vi "new_graph.vi"(4 "CurvesId":i32, 5 "D&T":string, 7 "connection ref":T1) -> (0 "error out":errorcluster, 1 "Waveform Graph":cluster{sgl, sgl, sgl[]}, 2 "reason":string, 3 "phwnd":string[][](table))   [LabVIEW 2010]
uses:
  <vilib>/addons/database/Connection.llb/Conn ObjectReference.ctl
  <vilib>/addons/database/NI_Database_API.lvlib
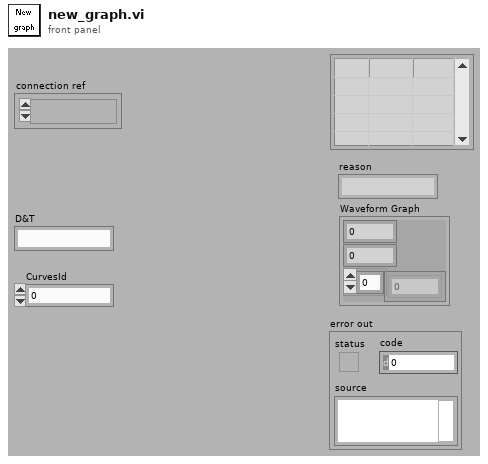
[diagram p1: front panel]
types:
  T1 = typedef "NI_Database_API.lvlib/Conn ObjectReference.ctl" = refnum<k1>
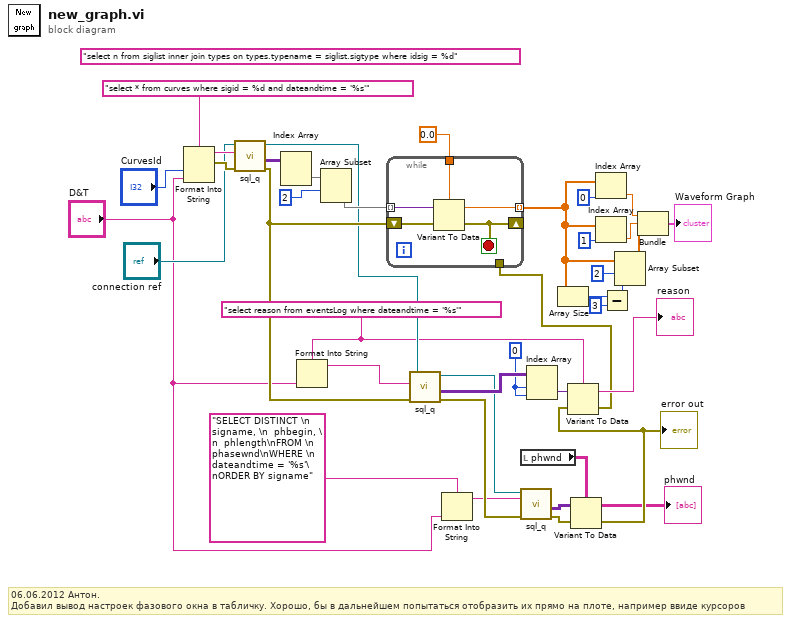
[diagram p0: block diagram]
diagram:
  w16 = 0 ("index (row)")
  w15 = "select reason from eventsLog where dateandtime = '%s'"
  (unwired) "select n from siglist inner join types on types.typename = siglist.sigtype where idsig = %d" ("regular expression (\"\")")
  # "06.06.2012 Антон. \nДобавил вывод настроек фазового окна в табличку. Хорошо, бы в дальнейшем попытаться отобразить их прямо на плоте, например ввиде курсоров"
  n1 = Format Into String(format string="select * from curves where sigid = %d and dateandtime = '%s'" ("optional clause"), "CurvesId", "D&T") -> (resulting string=w32:string, error out=w27:errorcluster)  [unwired: 2 in]
  n2 = call "sql_q.vi"("error in"=w27, "SQL query"=w32, "connect ref"="connection ref") -> ("error out"=w20:errorcluster, "recordset data"=w34:variant[][], "conn ref out"=w19:T1)  [unwired: 1 in, 1 out]
  n3 = Index Array(array=w34) -> (element=w35:variant[])  [unwired: 2 in]
  n4 = Format Into String(format string=w15, "D&T") -> (resulting string=w9:string)  [unwired: 2 in, 1 out]
  n5 = Array Subset(array=w35, index=2) -> (w33:variant[])  [unwired: 1 in]
  n6 = call "sql_q.vi"("error in"=w20, "SQL query"=w9, "connect ref"=w19) -> ("error out"=w11:errorcluster, "recordset data"=w18:variant[][], "conn ref out"=w6:T1)  [unwired: 1 in, 1 out]
  n7 = Format Into String(format string="SELECT DISTINCT \n  signame, \n  phbegin, \n  phlength\nFROM \n  phasewnd\nWHERE \n  dateandtime = '%s'\nORDER BY signame", "D&T") -> (resulting string=w7:string)  [unwired: 2 in, 1 out]
  n8 = local read "phwnd"() -> (w2:string[][])
  n9 = call "sql_q.vi"("error in"=w11, "SQL query"=w7, "connect ref"=w6) -> ("error out"=w4:errorcluster, "recordset data"=w5:variant[][])  [unwired: 1 in, 2 out]
  n10 = Index Array(array=w18, index (row)=w16, index (col)=w16) -> (element=w17:variant)
  n11 = Variant To Data(error in=w4, Variant=w5, type=w2) -> (error out=w3:errorcluster, data=→"phwnd":string[][])
  "error out" <- w3
  n12 = Variant To Data(error in=w3, Variant=w17, type=w15) -> (error out=w13:errorcluster, data=→"reason":string)
  n13 = while {
    tunnel: [w45] -> w23 mode=indexing
    tunnel: w33 -> [w44] mode=indexing
    shift-right: [w43] -> _
    shift-left: w20 -> [w42]
    tunnel: w13 -> [_]
    tunnel: 0.0 -> [w41]
    stop <- w43 stop-if-true
    n14 = Variant To Data(error in=w42, Variant=w44, type=w41) -> (error out=w43:errorcluster, data=w45:dbl)
  }
  n15 = Array Size(array=w23) -> (size(s)=w24:i32)
  n16 = Index Array(array=w23, index=0 ("disabled index (col)")) -> (element=w30:dbl)
  n17 = Index Array(array=w23, index=1 ("disabled index (col)")) -> (element=w31:dbl)
  n18 = Subtract(x=w24, y=3) -> (x-y=w22:i32)
  n19 = Array Subset(array=w23, index=2, length=w22) -> (w39:dbl[])
  n20 = Bundle(w30, w31, w39) -> (→"Waveform Graph":cluster{dbl, dbl, dbl[]})  [unwired: 1 in]
